vi "Msg.vi"(7 "Actor in":refnum<class "Actor.lvclass">, 11 "Msg in":refnum<class "Msg.lvclass">) -> (0 "Error out":errorcluster, 5 "Actor out":refnum<class "Actor.lvclass">)   [LabVIEW 2025, in "jettl.lvlib" / "Msg.lvclass"]
uses:
  Msg.lvclass
  Actor/Actor/Actor.lvclass
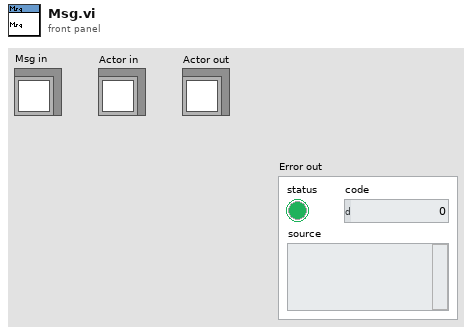
[diagram p1: front panel]
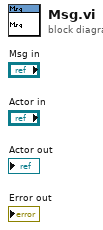
[diagram p0: block diagram]
diagram:
